vi "SubVI_StaticCharasteristic_YT.vi"(6 "Kvc":dbl, 7 "Tc":dbl, 8 "U":dbl[](array[numeric]), 9 "Kt":dbl, 10 "Te":dbl, 11 "Qe":dbl) -> (2 "Output":cluster{"U":dbl[], "Yt":dbl[]})   [LabVIEW 2020]
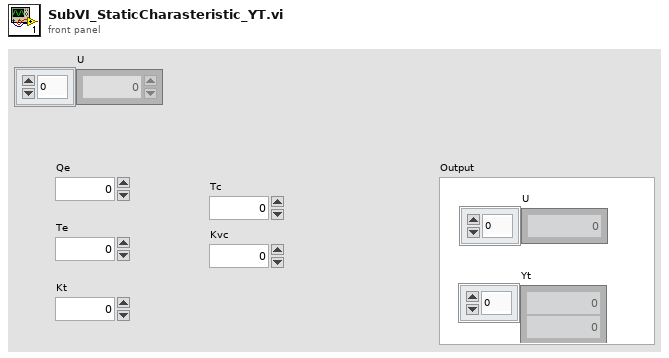
[diagram p1: front panel]
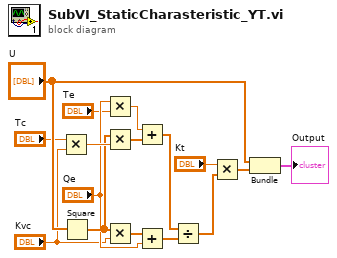
[diagram p0: block diagram]
diagram:
  n1 = Multiply(x="Tc", y="Kvc") -> (x*y=w15:dbl)
  n2 = Square(x="U") -> (x^2=w12:dbl[])
  n3 = Multiply(x="Qe", y="Te") -> (x*y=w14:dbl)
  n4 = Multiply(x=w12, y=w15) -> (x*y=w13:dbl[])
  n5 = Multiply(x=w12, y="Kvc") -> (x*y=w11:dbl[])
  n6 = Add(x=w14, y=w13) -> (x+y=w10:dbl[])
  n7 = Add(x=w11, y="Qe") -> (x+y=w9:dbl[])
  n8 = Divide(x=w10, y=w9) -> (x/y=w8:dbl[])
  n9 = Multiply(x="Kt", y=w8) -> (x*y=w7:dbl[])
  n10 = Bundle("U"="U", w7) -> (→"Output":cluster{"U":dbl[], dbl[]})  [unwired: 1 in]
